vi "_TextBoxLogCtrlMgr.Example.vi"() -> ()   [LabVIEW 2024, in "EQMF.lvlib" / "String Utils.lvlib"]
uses:
  String Utils.lvlib
  TextBoxLogCtrlMgr.lvclass
panel:
  in  "Clear":bool
  in  "Exit":bool
  in  "Re-Init":bool
  in  "Add Data":bool
  in  "New Data":string
  out "Log":string
  in  "Len":i32=200
  in  "Time En":bool
  in  "Date En":bool
  in  "Auto Scroll":bool
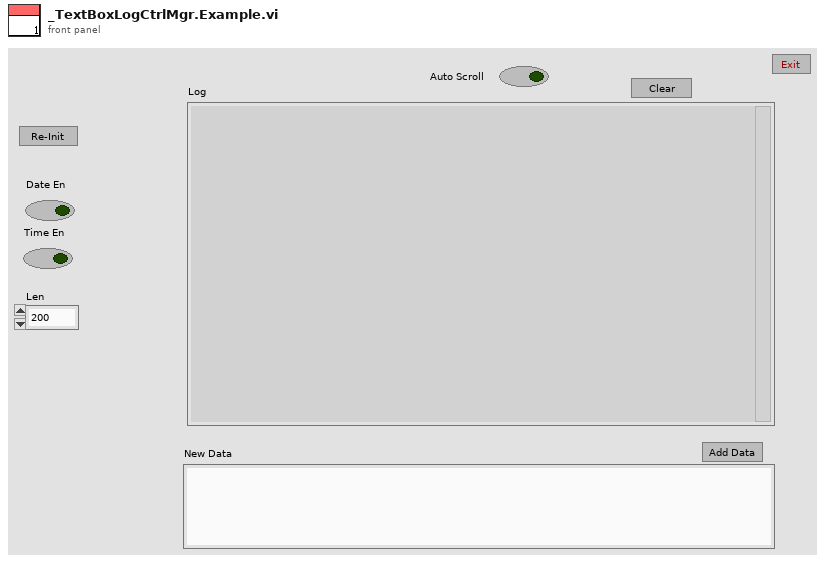
[diagram p1: front panel]
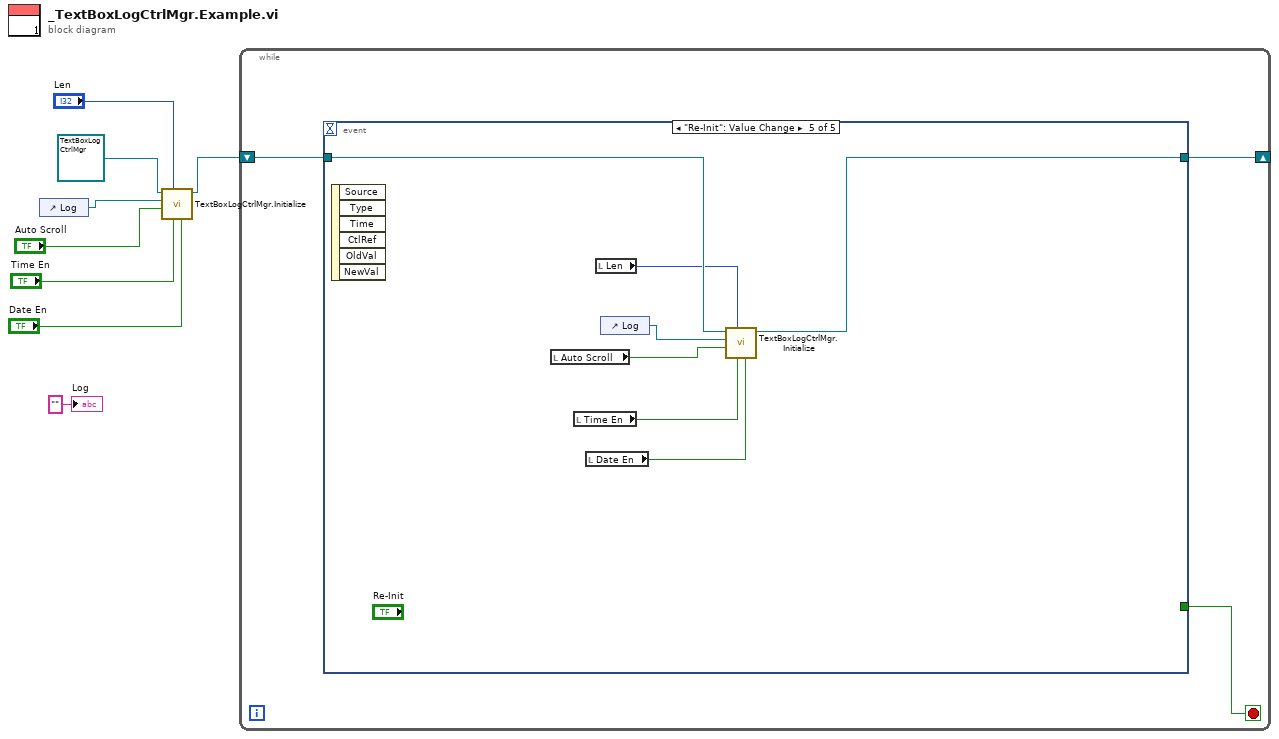
[diagram p0: block diagram]
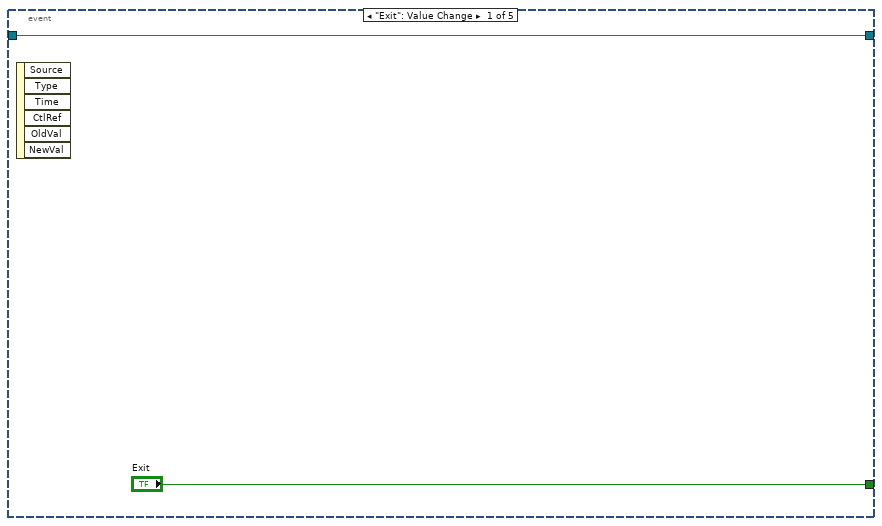
[diagram p2: hidden frame]
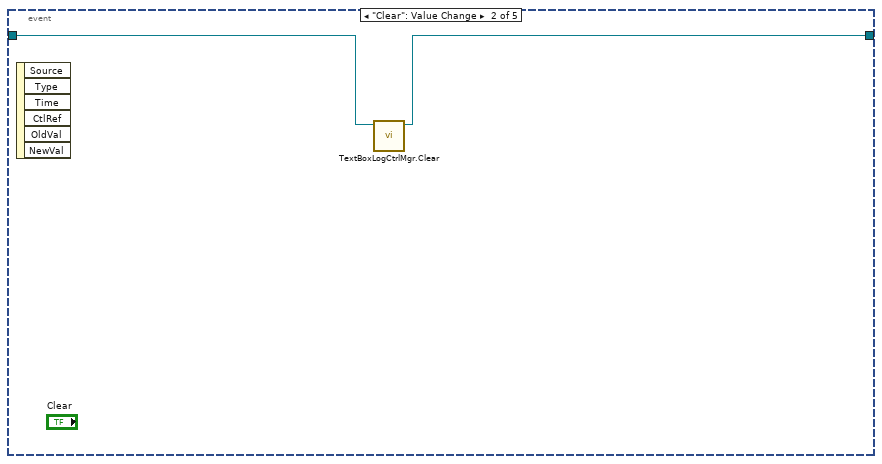
[diagram p3: hidden frame]
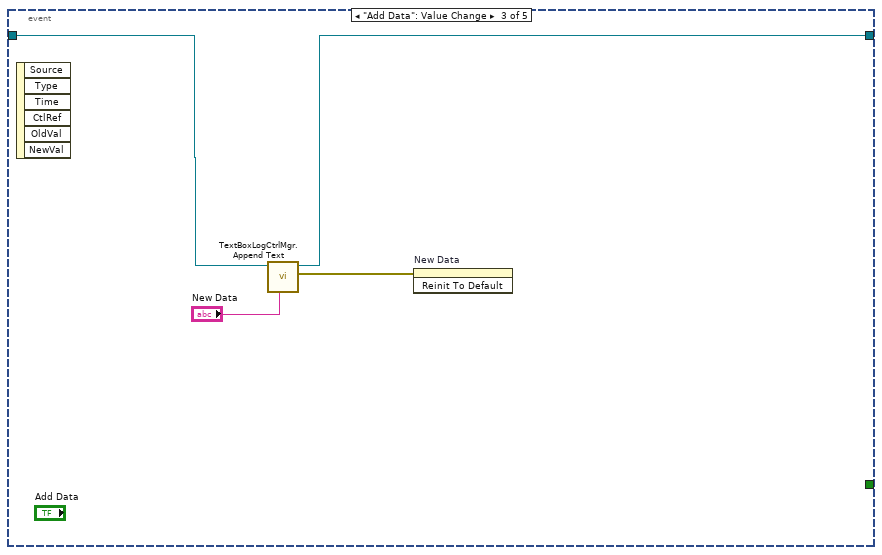
[diagram p4: hidden frame]
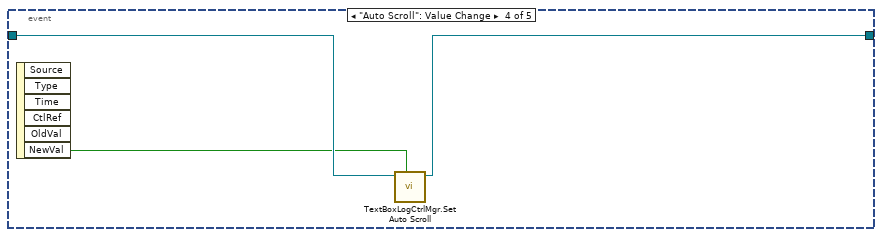
[diagram p5: hidden frame]
diagram:
  n1 = control-ref of="Log"() -> (w6:refnum<vi>)
  n2 = call "TextBoxLogCtrlMgr.Initialize.vi"("DataStamp"="Date En", "TimeStamp"="Time En", "MaxLen"="Len", "Auto Scroll"="Auto Scroll", "CtrlRef"=w6, "TextBoxLogCtrlMgr in"=refnum<class "TextBoxLogCtrlMgr.lvclass"> refnum ("KATE_Lib1:String Utils.lvlib:TextBoxLogCtrlMgr.lvclass")) -> ("TextBoxLogCtrlMgr out"=w7:refnum<class "TextBoxLogCtrlMgr.lvclass">)  [unwired: 4 in, 1 out]
  n3 = while {
    shift-right: [w10] -> _
    shift-left: w7 -> [w11]
    stop <- w9 stop-if-true
    n4 = event shown="[4] \"Re-Init\": Value Change" {
      selector: _ -> [_ _ _ _ _]
      dyn-events: _ -> [_ _ _ _ _]
      timeout: _ -> [_ _ _ _ _]
      tunnel: w11 -> [w13 w15 w19 w22 w25]
      tunnel: [w13 w14 w18 w21 w24] -> w10
      tunnel: ["Exit" _ _ _ _] -> w9
      event "Exit": Value Change {
        n5 = event-data() -> ()  [unwired: 1 in, 6 out]
      }
      event "Clear": Value Change {
        n6 = event-data() -> ()  [unwired: 1 in, 6 out]
        n7 = call "TextBoxLogCtrlMgr.Clear.vi"("TextBoxLogCtrlMgr in"=w15) -> ("TextBoxLogCtrlMgr out"=w14:refnum<class "TextBoxLogCtrlMgr.lvclass">)  [unwired: 9 in, 1 out]
      }
      event "Add Data": Value Change {
        n8 = event-data() -> ()  [unwired: 1 in, 6 out]
        n9 = call "TextBoxLogCtrlMgr.Append Text.vi"("Text In"="New Data", "TextBoxLogCtrlMgr in"=w19) -> ("error out"=w16:errorcluster, "TextBoxLogCtrlMgr out"=w18:refnum<class "TextBoxLogCtrlMgr.lvclass">)  [unwired: 8 in]
        n10 = invoke on="New Data" class="Str" method="Reinit To Default"(error in=w16) -> ()  [unwired: 2 in, 3 out]
      }
      event "Auto Scroll": Value Change {
        n11 = event-data() -> ("NewVal"=w20:bool)  [unwired: 1 in, 5 out]
        n12 = call "TextBoxLogCtrlMgr.Set Auto Scroll.vi"("Auto Scroll"=w20, "TextBoxLogCtrlMgr in"=w22) -> ("TextBoxLogCtrlMgr out"=w21:refnum<class "TextBoxLogCtrlMgr.lvclass">)  [unwired: 8 in, 1 out]
      }
      event "Re-Init": Value Change {
        n13 = event-data() -> ()  [unwired: 1 in, 6 out]
        n14 = local read "Auto Scroll"() -> (w27:bool)
        n15 = local read "Time En"() -> (w29:bool)
        n16 = local read "Date En"() -> (w28:bool)
        n17 = local read "Len"() -> (w23:i32)
        n18 = control-ref of="Log"() -> (w26:refnum<vi>)
        n19 = call "TextBoxLogCtrlMgr.Initialize.vi"("DataStamp"=w28, "TimeStamp"=w29, "MaxLen"=w23, "Auto Scroll"=w27, "CtrlRef"=w26, "TextBoxLogCtrlMgr in"=w25) -> ("TextBoxLogCtrlMgr out"=w24:refnum<class "TextBoxLogCtrlMgr.lvclass">)  [unwired: 4 in, 1 out]
      }
    }
  }
  "Log" <- "" ("Log")
